vi "Phasor Compute Calibrated SDV [(g, s) cal].vi"(8 "Error In":errorcluster, 9 "Phasor Calibration (g,s)":T1, 11 "Raw Phasor SDV (g, s)":T1) -> (0 "Error Out":errorcluster, 3 "Calibrated Phasor SDV (g, s)":T1)   [LabVIEW 2021, in "Phasor.lvlib"]
uses:
  Phasor.lvlib
  Phasor (g, s).ctl
panel:
  # "see the License on the block diagram (Ctrl+E or Window:Show Block Diagram)"
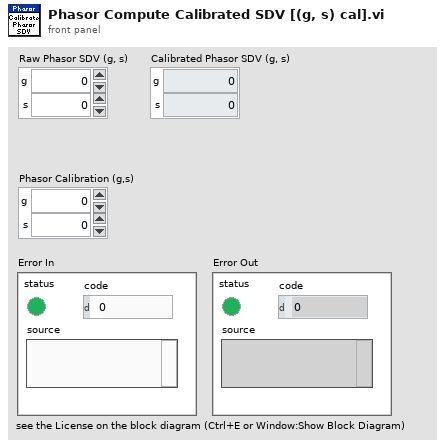
[diagram p1: front panel]
types:
  T1 = typedef "Phasor.lvlib/Phasor (g, s).ctl" = cluster{"g":dbl, "s":dbl}
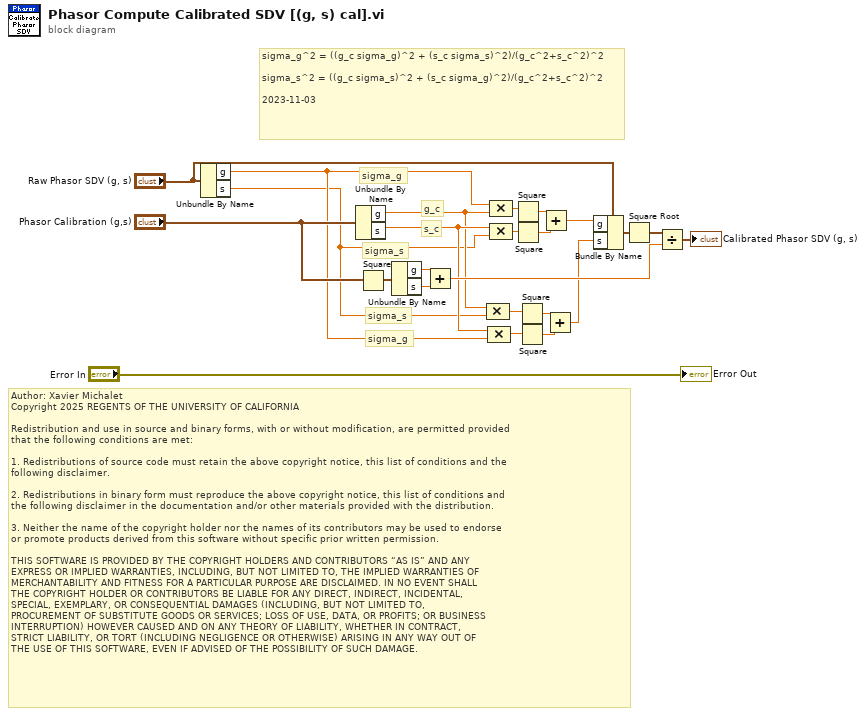
[diagram p0: block diagram]
diagram:
  # "Author: Xavier Michalet\nCopyright 2025 REGENTS OF THE UNIVERSITY OF CALIFORNIA\n\nRedistribution and use in source and binary forms, with or without modification, are permitted provided\nthat the following conditions are met:\n\n1. Redistributions of source code must retain the above copyright notice, this list of conditions and the\nfollowing disclaimer.\n\n2. Redistributions in binary form must reproduce the above copyright notice, this list of conditions and\nthe following disclaimer in the documentation and/or other materials provided with the distribution.\n\n3. Neither the name of the copyright holder nor the names of its contributors may be used to endorse \nor promote products derived from this software without specific prior written permission.\n\nTHIS SOFTWARE IS PROVIDED BY THE COPYRIGHT HOLDERS AND CONTRIBUTORS “AS IS” AND ANY \nEXPRESS OR IMPLIED WARRANTIES, INCLUDING, BUT NOT LIMITED TO, THE IMPLIED WARRANTIES OF\nMERCHANTABILITY AND FITNESS FOR A PARTICULAR PURPOSE ARE DISCLAIMED. IN NO EVENT SHALL\nTHE COPYRIGHT HOLDER OR CONTRIBUTORS BE LIABLE FOR ANY DIRECT, INDIRECT, INCIDENTAL, \nSPECIAL, EXEMPLARY, OR CONSEQUENTIAL DAMAGES (INCLUDING, BUT NOT LIMITED TO, \nPROCUREMENT OF SUBSTITUTE GOODS OR SERVICES; LOSS OF USE, DATA, OR PROFITS; OR BUSINESS\nINTERRUPTION) HOWEVER CAUSED AND ON ANY THEORY OF LIABILITY, WHETHER IN CONTRACT, \nSTRICT LIABILITY, OR TORT (INCLUDING NEGLIGENCE OR OTHERWISE) ARISING IN ANY WAY OUT OF\nTHE USE OF THIS SOFTWARE, EVEN IF ADVISED OF THE POSSIBILITY OF SUCH DAMAGE."
  # "sigma_g^2 = ((g_c sigma_g)^2 + (s_c sigma_s)^2)/(g_c^2+s_c^2)^2\n\nsigma_s^2 = ((g_c sigma_s)^2 + (s_c sigma_g)^2)/(g_c^2+s_c^2)^2\n\n2023-11-03"
  # "s_c"
  # "g_c"
  # "sigma_g"
  # "sigma_s"
  # "sigma_g"
  # "sigma_s"
  n1 = Unbundle By Name("Raw Phasor SDV (g, s)") -> ("g"=w2:dbl, "s"=w1:dbl)
  n2 = Unbundle By Name("Phasor Calibration (g,s)") -> ("g"=w13:dbl, "s"=w14:dbl)
  n3 = Square(x="Phasor Calibration (g,s)") -> (x^2=w10:T1)
  n4 = Unbundle By Name(w10) -> ("g"=w11:dbl, "s"=w12:dbl)
  n5 = Add(x=w11, y=w12) -> (x+y=w22:dbl)
  n6 = Compound Arithmetic op=MULTIPLY(w13, w1) -> (w17:dbl)
  n7 = Compound Arithmetic op=MULTIPLY(w14, w2) -> (w18:dbl)
  n8 = Compound Arithmetic op=MULTIPLY(w2, w13) -> (w6:dbl)
  n9 = Compound Arithmetic op=MULTIPLY(w14, w1) -> (w7:dbl)
  n10 = Square(x=w6) -> (x^2=w8:dbl)
  n11 = Square(x=w7) -> (x^2=w9:dbl)
  n12 = Square(x=w17) -> (x^2=w16:dbl)
  n13 = Square(x=w18) -> (x^2=w15:dbl)
  n14 = Add(x=w8, y=w9) -> (x+y=w19:dbl)
  n15 = Add(x=w16, y=w15) -> (x+y=w20:dbl)
  n16 = Bundle By Name(cluster="Raw Phasor SDV (g, s)", "g"=w19, "s"=w20) -> (w5:T1)
  n17 = Square Root(x=w5) -> (sqrt(x)=w21:T1)
  n18 = Divide(x=w21, y=w22) -> (x/y=→"Calibrated Phasor SDV (g, s)":T1)
  "Error Out" <- "Error In"
